vi "Event handler-AOL Z button.vi"(11 "AOL Z button's value":bool) -> (0 "error out":errorcluster)   [LabVIEW 2017]
uses:
  Typedefs/Set Main VI cursor.ctl
  Typedefs/Top level VI states.ctl
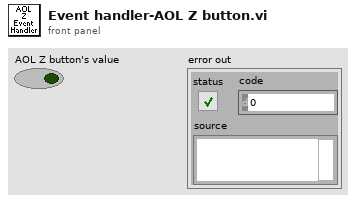
[diagram p1: front panel]
types:
  T1 = typedef "Set Main VI cursor.ctl" = enum16{"Release busy cursor", "Set busy cursor"}
  T2 = typedef "Top level VI states.ctl" = enum16{"None", "Initialise UI", "<STACK PROTOCOL STATES>", "AOL Zstack-START", "AOL Zstack-STOP", "Motor Zstack-START", "Motor Zstack-STOP", "<ACQUISITION PROTOCOL STATES> ", "Functional Acquisition-START", "Functional Acquisition-STOP", "Single Plane Acquisition-START", "Single Plane Acquisition-STOP", "Volume Acquisition-START", "Volume Acquisition-STOP", "<LIVE IMAGING PROTOCOL STATES>", "Live Imaging-START", "Live Imaging-STOP", "Live Plane Imaging-START", "Live Plane Imaging-STOP", "Live Volume Imaging-START", "Live Volume Imaging-STOP", "<MOVEMENT CORRECTION PROTOCOL STATES>", "Background MovCor-START", "Background MovCor-STOP", "EXIT"}
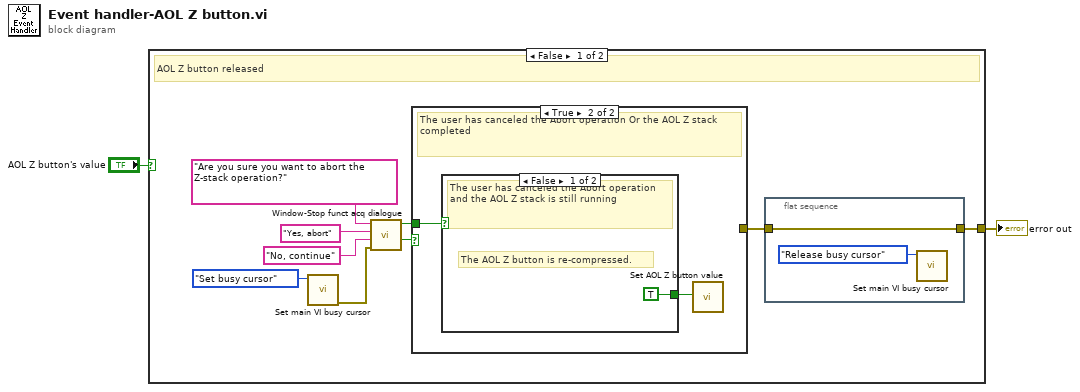
[diagram p0: block diagram]
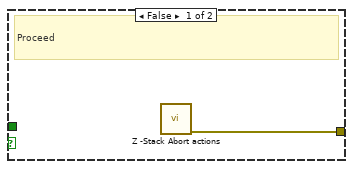
[diagram p2: hidden frame]
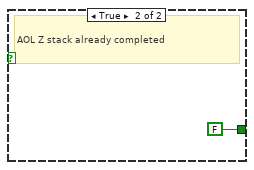
[diagram p3: hidden frame]
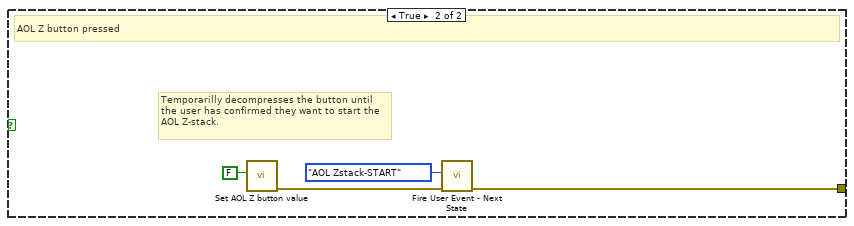
[diagram p4: hidden frame]
diagram:
  n1 = case shown="False" "AOL Z button's value" {
    tunnel: [w3 w20] -> w1
    frame False {
      # "AOL Z button released"
      n2 = call "Set main VI busy cursor.vi"("Main VI's cursor"=Set_Main_VI_cursor."Set busy cursor") -> ("error out"=w6:errorcluster)  [unwired: 10 in]
      n3 = call "Window-Stop funct acq dialogue.vi"("error in (no error)"=w6, "Caption-Left button (Cancel)"="No, continue", "Caption-Right button (OK)"="Yes, abort", "Message string"="Are you sure you want to abort the Z-stack operation?") -> ("User canceled the Abort Or the func acqcompleted"=w11:bool, "Funct acq completed"=w7:bool)  [unwired: 5 in, 1 out]
      n4 = case shown="True" w11 {
        tunnel: [w14 _] -> w4
        tunnel: w7 -> [_ w16]
        frame False {
          # "Proceed"
          n5 = call "Z -Stack Abort actions.vi"() -> ("error out"=w14:errorcluster)  [unwired: 11 in]
        }
        frame True {
          # "The user has canceled the Abort operation Or the AOL Z stack completed"
          n6 = case shown="False" w16 {
            tunnel: [TRUE ("Value") FALSE ("Value")] -> w15
            frame False {
              # "The AOL Z button is re-compressed."
              # "The user has canceled the Abort operation and the AOL Z stack is still running"
            }
            frame True {
              # "AOL Z stack already completed"
            }
          }
          n7 = call "Set AOL Z button value.vi"("AOL Z button's new value"=w15) -> ()  [unwired: 10 in, 1 out]
        }
      }
      n8 = flat-sequence {
        tunnel: w4 -> [w12]
        tunnel: [w12] -> w3
        frame #0 {
          n9 = call "Set main VI busy cursor.vi"("Main VI's cursor"=Set_Main_VI_cursor."Release busy cursor") -> ()  [unwired: 10 in, 1 out]
        }
      }
    }
    frame True {
      # "Temporarilly decompresses the button until the user has confirmed they want to start the AOL Z-stack."
      # "AOL Z button pressed"
      n10 = call "Set AOL Z button value.vi"("AOL Z button's new value"=FALSE ("Value")) -> ("error out"=w19:errorcluster)  [unwired: 10 in]
      n11 = call "Fire User Event - Next State.vi"("Error In"=w19, "\"UI Handler loop\" case to execute"=Top_level_VI_states."AOL Zstack-START" ("event data / imaging mode")) -> ("Error Out"=w20:errorcluster)  [unwired: 9 in]
    }
  }
  "error out" <- w1
